vi "AutoMatch.vi"() -> ()   [LabVIEW 2015]
panel:
  out "Current Iteretions":i32
  out "Current Numeric":dbl format="%#.0f"
  in  "Numeric":u32=50 max=1000 step=1
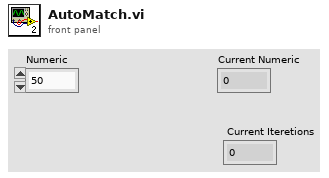
[diagram p1: front panel]
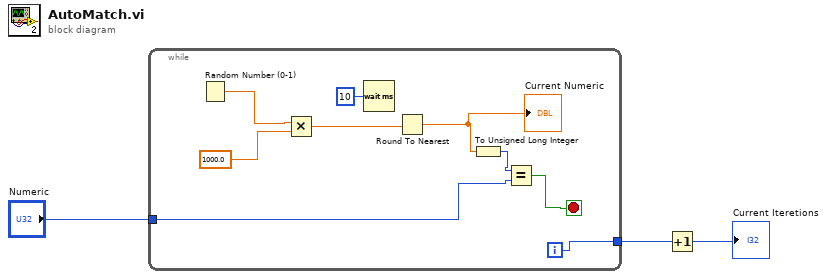
[diagram p0: block diagram]
diagram:
  n1 = while {
    tunnel: "Numeric" -> [w9]
    tunnel: [w8] -> w2
    i -> [w8]
    stop <- w7 stop-if-true
    n2 = Random Number (0-1)() -> (number: 0 to 1=w12:dbl)
    n3 = Multiply(x=w12, y=1000.0) -> (x*y=w10:dbl)
    n4 = Wait (ms)(milliseconds to wait=u32 10) -> ()  [unwired: 1 out]
    n5 = Round To Nearest(number=w10) -> (nearest integer value=w5:dbl)
    "Current Numeric" <- w5
    n6 = To Unsigned Long Integer(number=w5) -> (unsigned 32bit integer=w4:u32)
    n7 = Equal?(x=w4, y=w9) -> (x = y?=w7:bool)
  }
  n8 = Increment(x=w2) -> (x+1=→"Current Iteretions":i32)
